vi "Status Get Flow Rate.vi"(5 "Retry Attempts (0)":i32 min=0, 7 "Fast Comms (F)":bool, 8 "error in":errorcluster, 11 "VISA resource name":refnum<visa-resource-name>) -> (0 "error out":errorcluster, 2 "Flow Rate":dbl, 3 "VISA resource name out":refnum<visa-resource-name>)   [LabVIEW 2020, in "ChromTech MX-Class Drivers.lvlib"]
doc: "Query the pump for the current flow rate."
uses:
  ChromTech MX-Class Drivers.lvlib
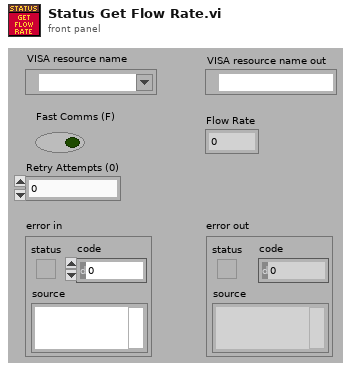
[diagram p1: front panel]
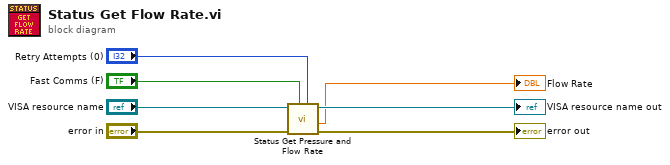
[diagram p0: block diagram]
diagram:
  n1 = call "Status Get Pressure and Flow Rate.vi"("Retry Attempts (0)"="Retry Attempts (0)", "Fast Comms (F)"="Fast Comms (F)", "error in"="error in", "VISA resource name"="VISA resource name") -> ("error out"=→"error out":errorcluster, "Flow Rate"=→"Flow Rate":dbl, "VISA resource name out"=→"VISA resource name out":refnum<visa-resource-name>)  [unwired: 4 in, 1 out]
